vi "Update Summary.vi"(8 "error in (no error)":errorcluster, 9 "Error Status":bool, 10 "Level":T1=enum."Info", 11 "Event Reporter Module in":refnum<class "Event Reporter Module.lvclass">) -> (0 "error out":errorcluster, 3 "Event Reporter Module out":refnum<class "Event Reporter Module.lvclass">)   [LabVIEW 2020, in "Volatus.lvlib" / "Event Reporter Module.lvclass"]
uses:
  Event Reporter Module.lvclass
  Event Reporter Module.lvclass/Event Reporter Module.ctl
  Event Level.ctl
  Volatus.lvlib
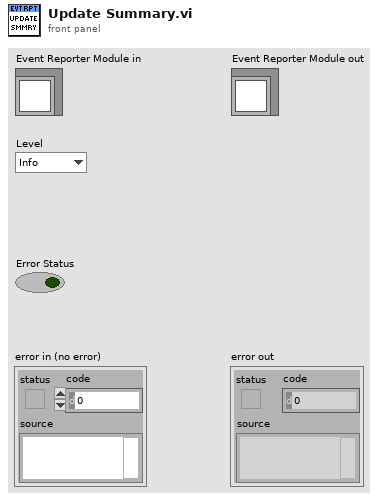
[diagram p1: front panel]
types:
  T1 = typedef "Volatus.lvlib/Event Level.ctl" = enum16{"Debug", "Info", "Warning", "Error"}
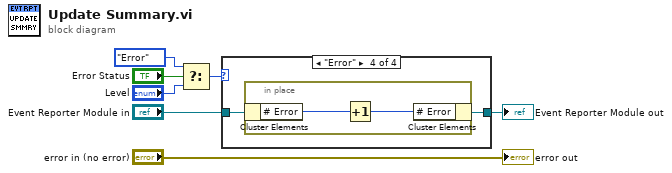
[diagram p0: block diagram]
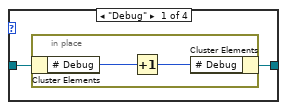
[diagram p2: hidden frame]
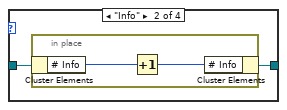
[diagram p3: hidden frame]
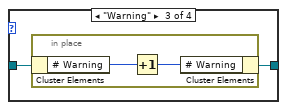
[diagram p4: hidden frame]
diagram:
  n1 = Select(t=Event_Level."Error", s="Error Status", f="Level") -> (s? t:f=w5:T1)
  n2 = case shown="\"Error\"" w5 {
    tunnel: "Event Reporter Module in" -> [w9 w13 w17 w21]
    tunnel: [w8 w12 w16 w20] -> w3
    frame "Debug" {
      n3 = in-place {
        n4 = in-place-cluster #1(w9) -> ("# Debug"=w11:i32)
        n5 = Increment(x=w11) -> (x+1=w10:i32)
        n6 = in-place-cluster #1("# Debug"=w10) -> (w8:refnum<class "Event Reporter Module.lvclass">)
      }
    }
    frame "Info" {
      n7 = in-place {
        n8 = in-place-cluster #2(w13) -> ("# Info"=w15:i32)
        n9 = Increment(x=w15) -> (x+1=w14:i32)
        n10 = in-place-cluster #2("# Info"=w14) -> (w12:refnum<class "Event Reporter Module.lvclass">)
      }
    }
    frame "Warning" {
      n11 = in-place {
        n12 = in-place-cluster #3(w17) -> ("# Warning"=w19:i32)
        n13 = Increment(x=w19) -> (x+1=w18:i32)
        n14 = in-place-cluster #3("# Warning"=w18) -> (w16:refnum<class "Event Reporter Module.lvclass">)
      }
    }
    frame "Error" {
      n15 = in-place {
        n16 = in-place-cluster #4(w21) -> ("# Error"=w23:i32)
        n17 = Increment(x=w23) -> (x+1=w22:i32)
        n18 = in-place-cluster #4("# Error"=w22) -> (w20:refnum<class "Event Reporter Module.lvclass">)
      }
    }
  }
  "Event Reporter Module out" <- w3
  "error out" <- "error in (no error)"
